vi "ADC_Running.vi"(8 "error in (no error)":errorcluster) -> (0 "error out":errorcluster, 3 "function return":i16)   [LabVIEW 2013, in "MeasurmentRoutines.lvlib"]
doc: "Description: This routine checks if the hardware is currently measuring\nInput: -\nOutput: Return value 0 = not measuring | 1 = measuring\n\nFunction prototype: word ADC_Running( void )\n\n\n\n\n\n\n\n\n\nshort int ADC_Running ( void );"
uses:
  MeasurmentRoutines.lvlib
  hs3.dll
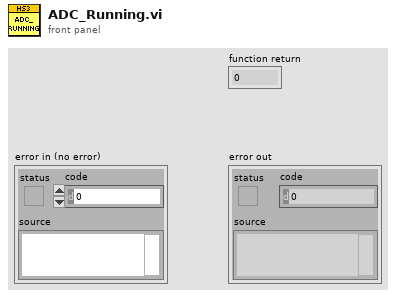
[diagram p1: front panel]
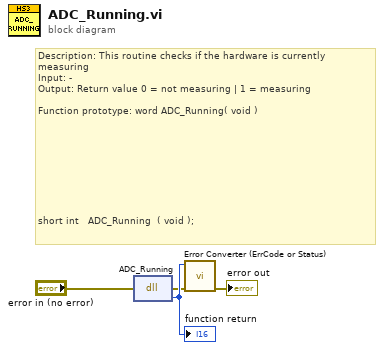
[diagram p0: block diagram]
diagram:
  # "Description: This routine checks if the hardware is currently measuring\nInput: -\nOutput: Return value 0 = not measuring | 1 = measuring\n\nFunction prototype: word ADC_Running( void )\n\n\n\n\n\n\n\n\n\nshort int \t\tADC_Running\t\t( void );"
  n1 = dll-call lib="C:/Documents and Settings/admin/Pulpit/HS3 LabViewLib/HS3_WRAPPER/hs3.*" fn="ADC_Running"(error in="error in (no error)") -> (error out=w2:errorcluster, w4:i16)  [unwired: 2 in, 1 out]
  "function return" <- w4
  n2 = call "Error Converter (ErrCode or Status).vi"("error in (no error)"=w2, "error code"=w4) -> ("error out"=→"error out":errorcluster)  [unwired: 9 in]
